vi "send_chart_data.vi"(8 "error in (no error)":errorcluster, 10 "getData":dbl[](array[numeric]), 11 "events":T1) -> (0 "error in (no error) 2":errorcluster, 3 "events 2":T1)   [LabVIEW 2018]
uses:
  swabian_events_tdef.ctl
  update_chart_tdef.ctl
  channel_data_tdef.ctl
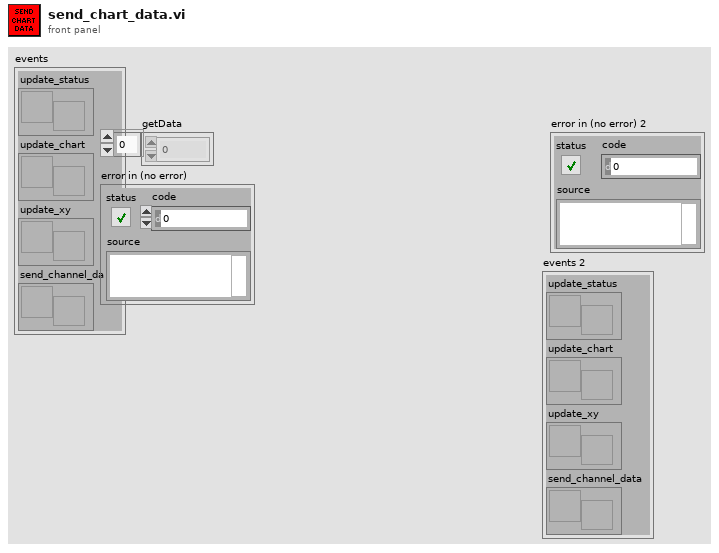
[diagram p1: front panel]
types:
  T1 = typedef "swabian_events_tdef.ctl" = cluster{"update_status":refnum<user-event>, "update_chart":refnum<user-event>, "update_xy":refnum<user-event>, "send_channel_data":refnum<user-event>}
  T2 = typedef "update_chart_tdef.ctl" = cluster{"ch0":dbl, "ch1":dbl, "ch2":dbl, "ch3":dbl, "ch4":dbl, "ch5":dbl, "ch6":dbl, "ch7":dbl}
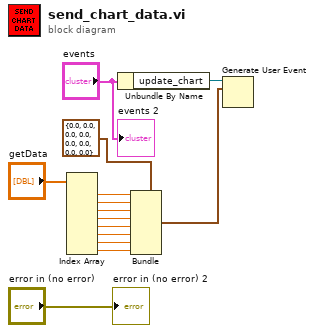
[diagram p0: block diagram]
diagram:
  n1 = Index Array(array="getData") -> (element #1=w10:dbl, element #2=w9:dbl, element #3=w8:dbl, element #4=w7:dbl, element #5=w6:dbl, element #6=w5:dbl, element #7=w4:dbl, element #8=w3:dbl)  [unwired: 8 in]
  n2 = Unbundle By Name("events") -> ("update_chart"=w13:refnum<user-event>)
  n3 = Bundle(cluster=T2 {"ch0"=0.0, "ch1"=0.0, "ch2"=0.0, "ch3"=0.0, "ch4"=0.0, "ch5"=0.0, "ch6"=0.0, "ch7"=0.0} ("event data"), "ch0"=w10, "ch1"=w9, "ch2"=w8, "ch3"=w7, "ch4"=w6, "ch5"=w5, "ch6"=w4, "ch7"=w3) -> (w2:T2)
  n4 = Generate User Event(user event=w13, event data cluster=w2) -> ()  [unwired: 2 in, 2 out]
  "error in (no error) 2" <- "error in (no error)"
  "events 2" <- "events"
